vi "Assert Less_Variant.vi"(4 "Execution time (s)":dbl=-1.0, 6 "error code (1)":i32=1, 7 "Label":string, 8 "error in":errorcluster, 10 "Y":variant, 11 "X":variant) -> (0 "error out":errorcluster, 2 "Properties":refnum<class "Properties.Assert.lvclass">)   [LabVIEW 2021, in "Banana.Caraya.lvlib" / "Platano.CarayaTestSuite.lvclass"]
uses:
  Platano.CarayaTestSuite.lvclass
  Platano.CarayaTestSuite.lvclass/Platano.CarayaTestSuite.ctl
  <vilib>/addons/_JKI Toolkits/Caraya/classes/Assert/Assert.lvclass
  Bananas/Platano/Platano.lvclass
  Bananas/Banana/Banana.lvclass
  Bananas/AssertCompareValue/AssertCompareValue.lvclass
  Leaf.Properties.Assert/Leaf.Properties.Assert.lvclass
  Bananas/Leaf/Leaf.lvclass
  C:/Repositories/LVOS/Bananas/lv-src/Banana.Caraya/Leaf.Properties/Leaf.Properties.lvclass
  C:/Program Files (x86)/National Instruments/LabVIEW 2021/vi.lib/addons/_JKI Toolkits/Caraya/classes/Properties/Properties.lvclass
  C:/Repositories/LVOS/Bananas/lv-src/Bananas/Leaf.Assertion/Leaf.Assertion.lvclass
  C:/Repositories/LVOS/Bananas/lv-src/Bananas/Leaf/Leaf.lvclass
  C:/Repositories/LVOS/Bananas/lv-src/Banana.Caraya/Leaf.Properties.Assert/Leaf.Properties.Assert.lvclass
  C:/Repositories/LVOS/Bananas/lv-src/Bananas/AssertCompareValue/AssertCompareValue.lvclass
  C:/Repositories/LVOS/Bananas/lv-src/Bananas/BananaPeel/BananaPeel.lvclass
  Bananas/Leaf.Assertion/Leaf.Assertion.lvclass
  <vilib>/addons/_JKI Toolkits/Caraya/classes/Properties.Assert/Properties.Assert.lvclass
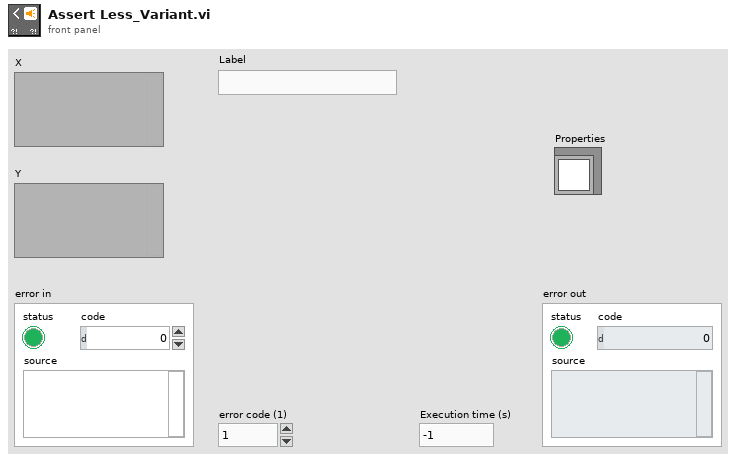
[diagram p1: front panel]
types:
  T1 = typedef "Bananas.lvlib/Assertion Strategies -- cluster.ctl" = cluster{"AssertTrue":refnum<class "AssertTrue.lvclass">, "AssertFalse":refnum<class "AssertFalse.lvclass">, "AssertEqualValue":refnum<class "AssertEqualValue.lvclass">, "AssertEqualType":refnum<class "AssertEqualType.lvclass">, "AssertCompareValue":refnum<class "AssertCompareValue.lvclass">, "AssertError":refnum<class "AssertError.lvclass">, "AssertAlmostEqual":refnum<class "AssertAlmostEqualValue.lvclass">}
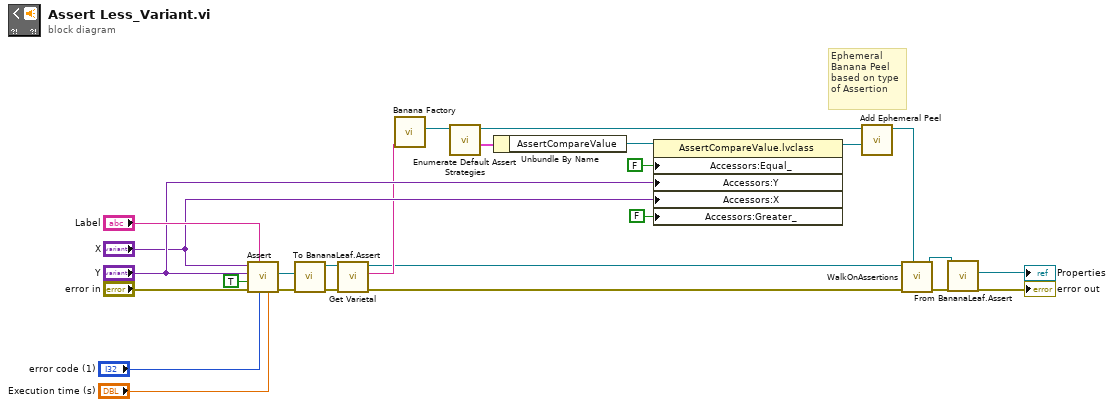
[diagram p0: block diagram]
diagram:
  # "Ephemeral\nBanana Peel\nbased on type\nof Assertion"
  n1 = call-poly <vilib>:"Assert.vi"("Execution time (s)"="Execution time (s)", "error code (1)"="error code (1)", "Label"="Label", "error in (no error)"="error in", "Register with caller test (F)"=TRUE, "Y"="Y", "X"="X") -> ("error out"=w3:errorcluster, "Properties.Assert"=w4:refnum<class "Properties.Assert.lvclass">)  [unwired: 3 in]
  n2 = call "To BananaLeaf.Assert.vi"("Properties.Assert"=w4) -> ("Leaf.Properties.Assert out"=w8:refnum<class "Leaf.Properties.Assert.lvclass">)  [unwired: 10 in]
  n3 = call "Get Varietal.vi"("error in (no error)"=w3, "Leaf in"=w8) -> ("error out"=w7:errorcluster, "Varietal"=w6:string, "Leaf out"=w5:refnum<class "Leaf.Properties.Assert.lvclass">)  [unwired: 7 in]
  n4 = call "Banana Factory.vi"("Varietal"=w6) -> ("Banana"=w9:refnum<class "Banana.lvclass">)  [unwired: 9 in, 1 out]
  n5 = call "Enumerate Default Assert Strategies.vi"("Banana"=w9) -> ("Strategies"=w13:T1, "Banana"=w17:refnum<class "Banana.lvclass">)  [unwired: 9 in]
  n6 = Unbundle By Name(w13) -> ("AssertCompareValue"=w16:refnum<class "AssertCompareValue.lvclass">)
  n7 = property class="AssertCompareValue.lvclass"(reference=w16, "Accessors:Equal_"=FALSE ("Equal_"), "Accessors:Y"="Y", "Accessors:X"="X", "Accessors:Greater_"=FALSE ("Greater_")) -> (reference out=w12:refnum<class "AssertCompareValue.lvclass">)  [unwired: 1 in, 1 out]
  n8 = call "Add Ephemeral Peel.vi"("BananaPeel"=w12, "Banana"=w17) -> ("Banana"=w18:refnum<class "Banana.lvclass">)  [unwired: 9 in]
  n9 = call "WalkOnAssertions.vi"("Banana"=w18, "error in (no error)"=w7, "Leaf.Assertion"=w5) -> ("error out"=→"error out":errorcluster, "Leaf.Assertion"=w2:refnum<class "Leaf.Assertion.lvclass">)  [unwired: 7 in]
  n10 = call "From BananaLeaf.Assert.vi"("Leaf.Properties.Assert"=w2) -> ("Properties.Assert"=→"Properties":refnum<class "Properties.Assert.lvclass">)  [unwired: 10 in]
